vi "Failed attempt Main_11b.vi"() -> ()   [LabVIEW 2020]
uses:
  4985a7b0-beb7-44e5-b21a-1b7cc2dea417.vi
  Cluster_Multiply.ctl
panel:
  out "Array":T1(array[cluster])
  out "Answer":i32
  in  "Puzzle":string="Monkey 0:\n  Starting items: 72, 97\n  Operation: new = old * 13\n  Test: divisible by 19\n    If true: throw to monkey 5\n    If false: throw to monkey 6\n\nMonkey 1:\n  Starting items: 55, 70, 90, 74, 95\n  Operation: new = old * old\n  Test: divisible by 7\n    If true: throw to monkey 5\n    If false: throw to monkey 0\n\nMonkey 2:\n  Starting items: 74, 97, 66, 57\n  Operation: new = old + 6\n  Test: divisible by 17\n    If true: throw to monkey 1\n    If false: throw to monkey 0\n\nMonkey 3:\n  Starting items: 86, 54, 53\n  Operation: new = old + 2\n  Test: divisible by 13\n    If true: throw to monkey 1\n    If false: throw to monkey 2\n\nMonkey 4:\n  Starting items: 50, 65, 78, 50, 62, 99\n  Operation: new = old + 3\n  Test: divisible by 11\n    If true: throw to monkey 3\n    If false: throw to monkey 7\n\nMonkey 5:\n  Starting items: 90\n  Operation: new = old + 4\n  Test: divisible by 2\n    If true: throw to monkey 4\n    If false: throw to monkey 6\n\nMonkey 6:\n  Starting items: 88, 92, 63, 94, 96, 82, 53, 53\n  Operation: new = old + 8\n  Test: divisible by 5\n    If true: throw to monkey 4\n    If false: throw to monkey 7\n\nMonkey 7:\n  Starting items: 70, 60, 71, 69, 77, 70, 98\n  Operation: new = old * 7\n  Test: divisible by 3\n    If true: throw to monkey 2\n    If false: throw to monkey 3"
  in  "Example":string="Monkey 0:\n  Starting items: 79, 98\n  Operation: new = old * 19\n  Test: divisible by 23\n    If true: throw to monkey 2\n    If false: throw to monkey 3\n\nMonkey 1:\n  Starting items: 54, 65, 75, 74\n  Operation: new = old + 6\n  Test: divisible by 19\n    If true: throw to monkey 2\n    If false: throw to monkey 0\n\nMonkey 2:\n  Starting items: 79, 60, 97\n  Operation: new = old * old\n  Test: divisible by 13\n    If true: throw to monkey 1\n    If false: throw to monkey 3\n\nMonkey 3:\n  Starting items: 74\n  Operation: new = old + 3\n  Test: divisible by 17\n    If true: throw to monkey 0\n    If false: throw to monkey 1"
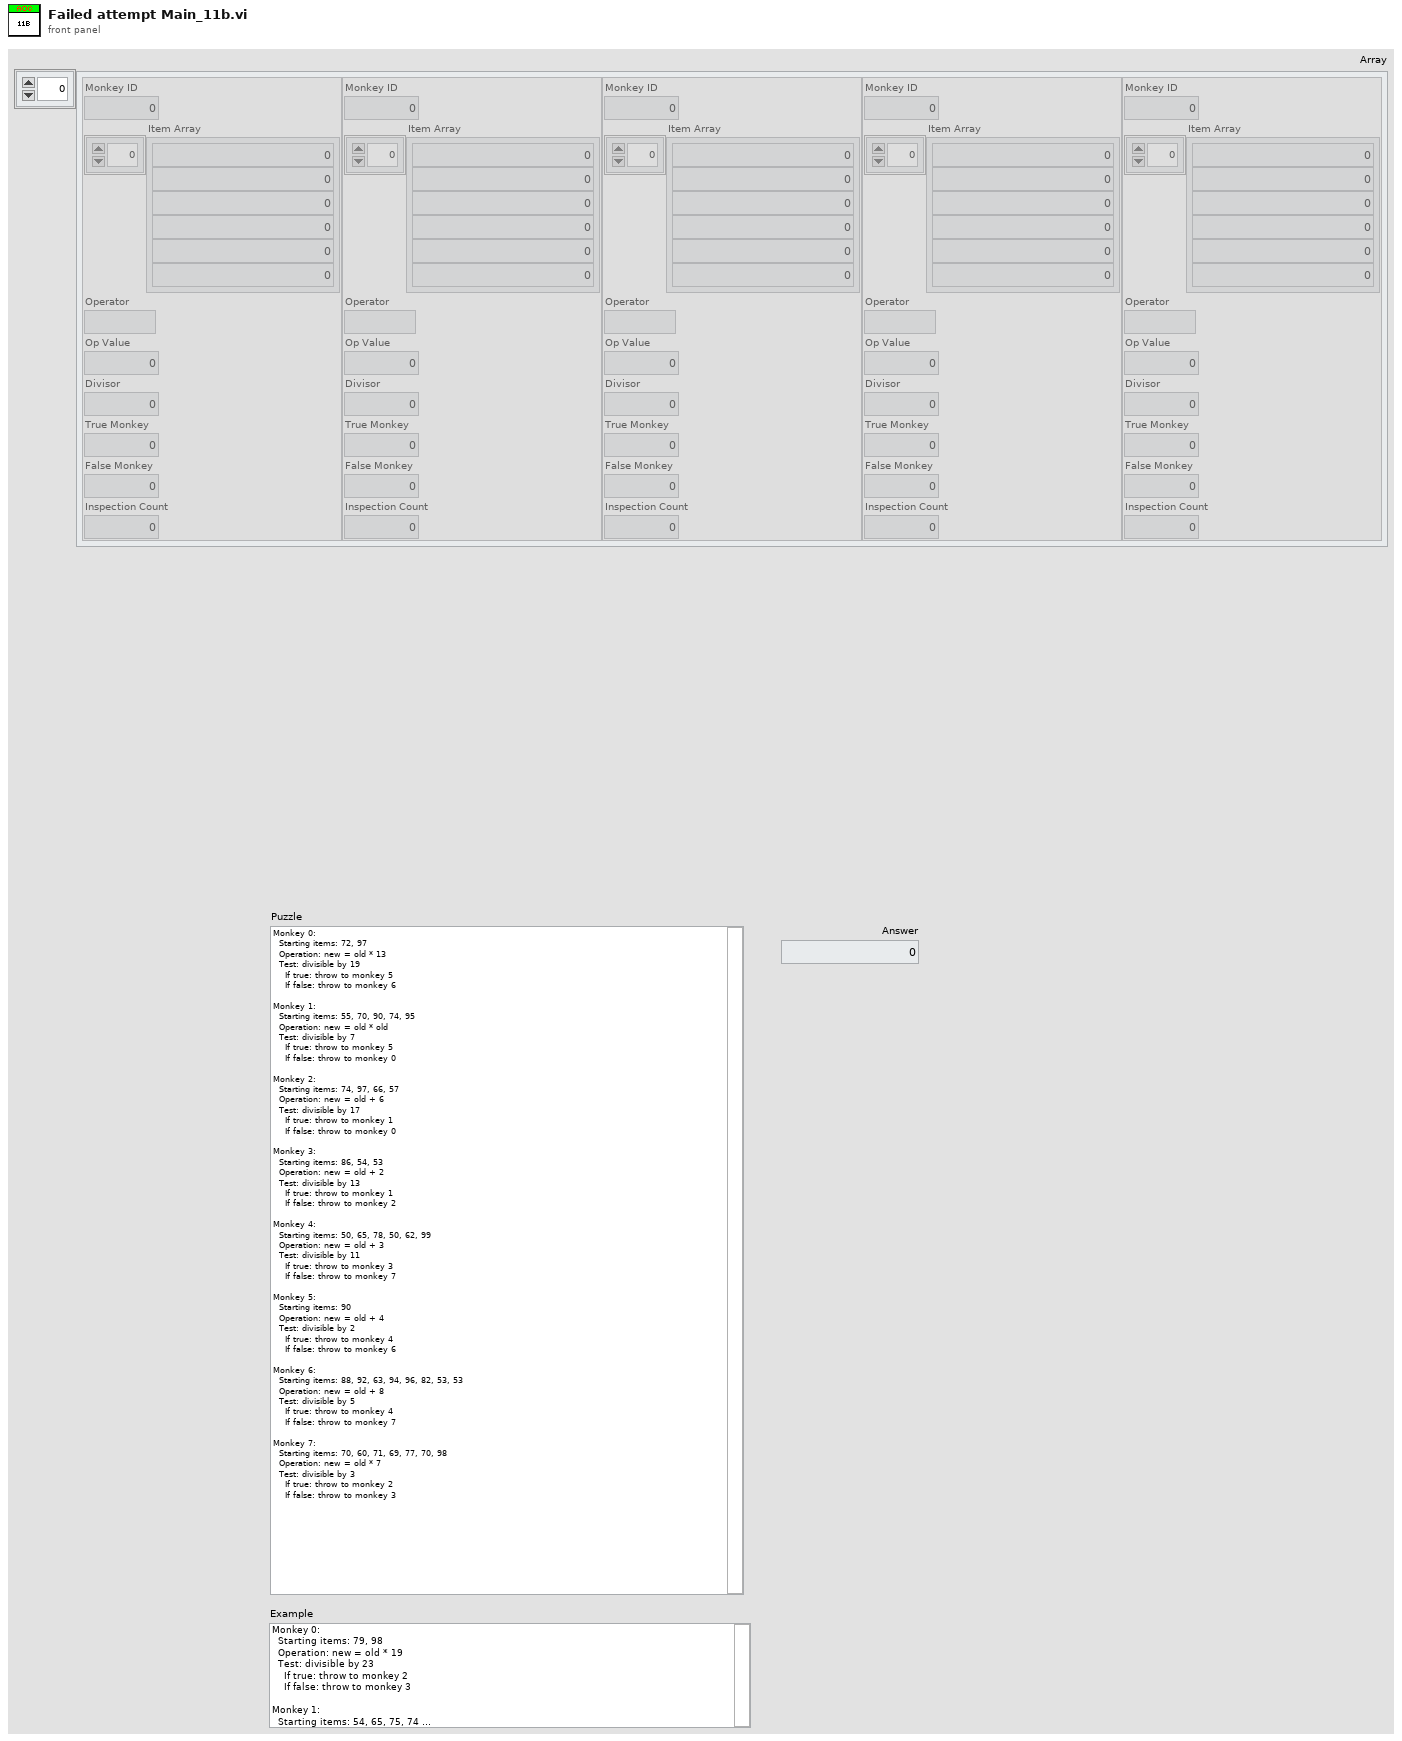
[diagram p1: front panel]
types:
  T1 = cluster{"Monkey ID":i32, "Item Array":u64[], "Operator":string, "Op Value":u64, "Divisor":u64, "True Monkey":i32, "False Monkey":i32, "Inspection Count":u64}[]
  T2 = typedef "Cluster_Multiply.ctl" = cluster{"Multiply Array":u64[]}
  T3 = cluster{"Monkey ID":i32, "Item":u64, "Operator":string, "Op Value":u64, "Divisor":u64, "True Monkey":i32, "False Monkey":i32, "Inspection Count":u64}
  T4 = cluster{"Monkey ID":i32, "Item":u64, "Operator":string, "Op Value":u64, "Divisor":u64, "True Monkey":i32, "False Monkey":i32, "Inspection Count":u64}[]
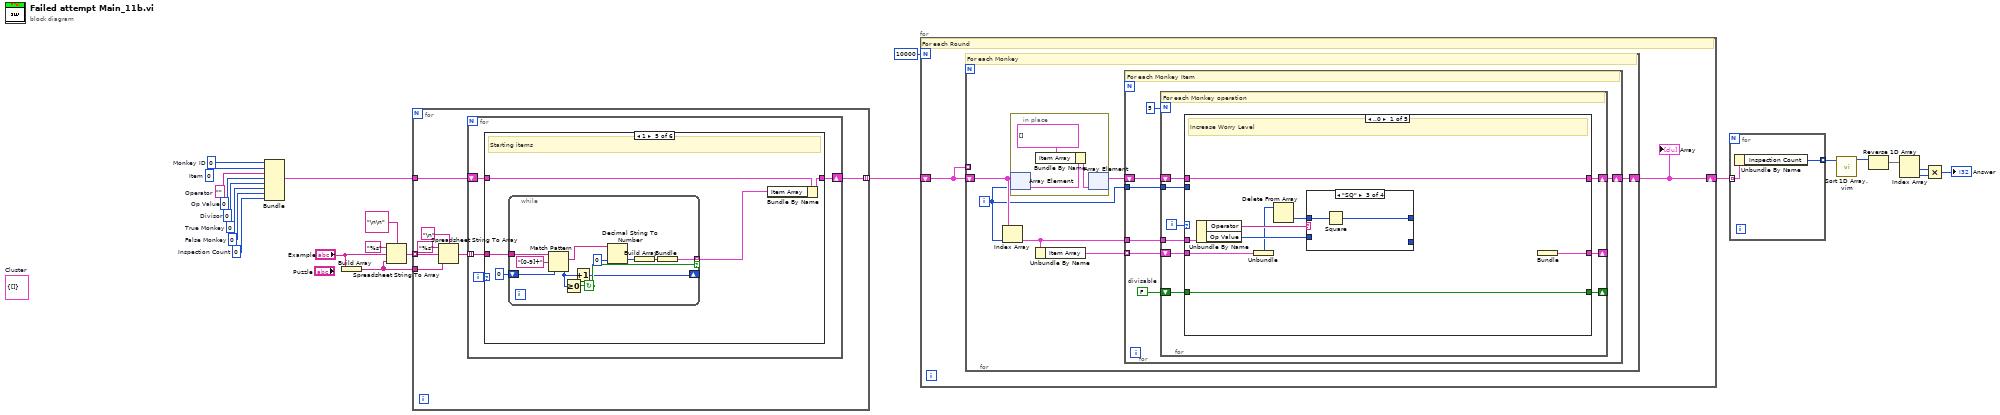
[diagram p0: block diagram]
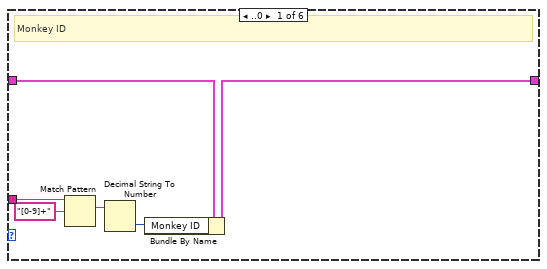
[diagram p2: hidden frame]
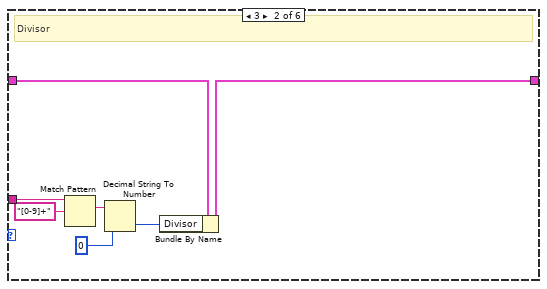
[diagram p3: hidden frame]
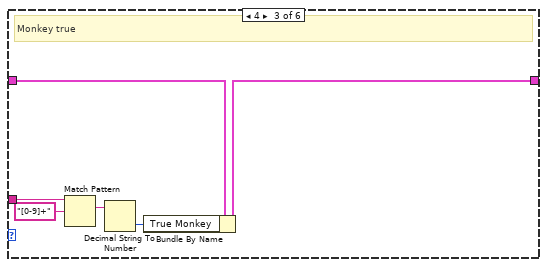
[diagram p4: hidden frame]
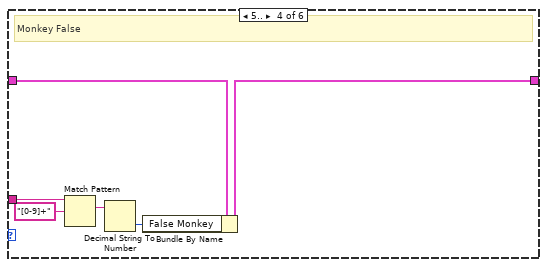
[diagram p5: hidden frame]
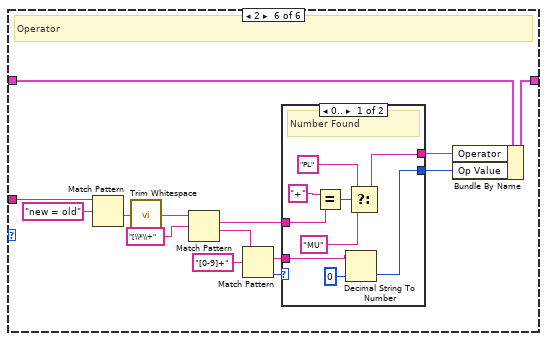
[diagram p6: hidden frame]
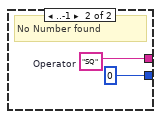
[diagram p7: hidden frame]
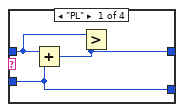
[diagram p8: hidden frame]
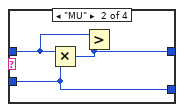
[diagram p9: hidden frame]
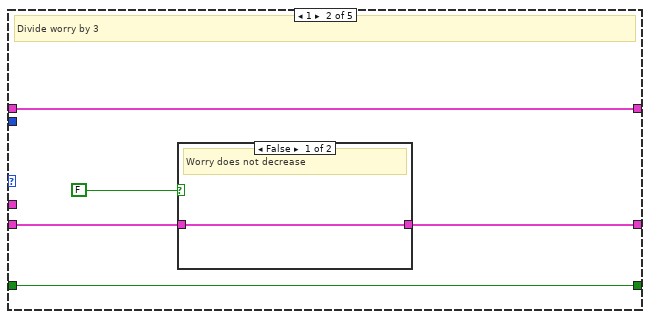
[diagram p11: hidden frame]
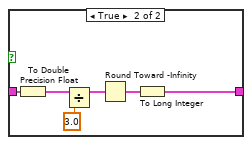
[diagram p12: hidden frame]
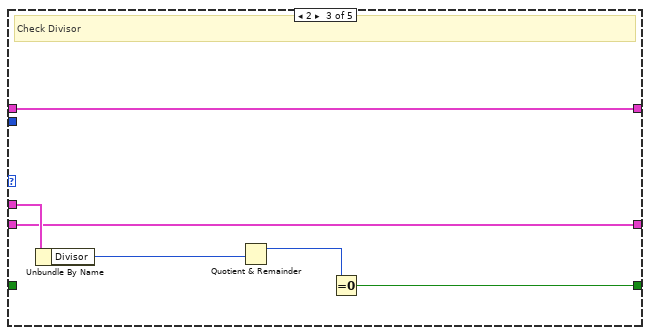
[diagram p13: hidden frame]
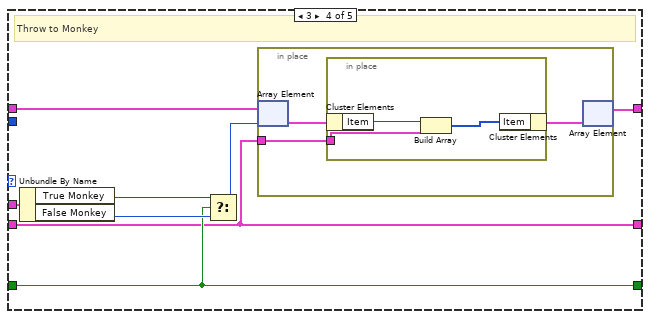
[diagram p14: hidden frame]
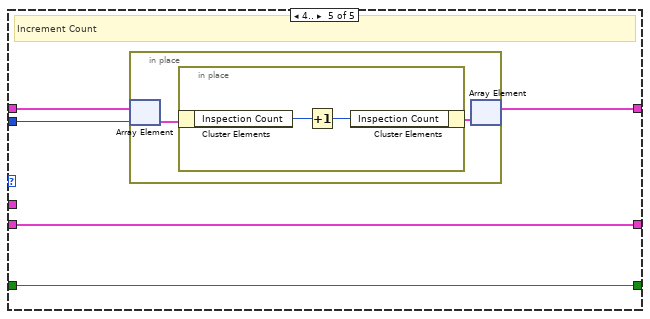
[diagram p15: hidden frame]
diagram:
  w1 = u64 0  # Item
  (unwired) T2 {"Multiply Array"=[]}  # Cluster
  w10 = u64 0  # Inspection Count
  w13 = 0  # False Monkey
  w14 = 0  # True Monkey
  w15 = u64 0  # Divisor
  w16 = u64 0  # Op Value
  w17 = ""  # Operator
  w18 = 0  # Monkey ID
  n1 = Bundle("Monkey ID"=w18, "Item"=w1, "Operator"=w17, "Op Value"=w16, "Divisor"=w15, "True Monkey"=w14, "False Monkey"=w13, "Inspection Count"=w10) -> (w12:T3)  [unwired: 1 in]
  n2 = Build Array("Example") -> (w19:string[])
  n3 = Spreadsheet String To Array(delimiter (Tab)="\n\n", format string="%s", spreadsheet string="Example", array type (2D Dbl)=w19) -> (array=w20:string[])
  n4 = for {
    tunnel: w20 -> [w30] mode=indexing
    tunnel: w19 -> [w27]
    tunnel: w12 -> [w25]
    tunnel: [w24] -> w11 mode=indexing
    n5 = Spreadsheet String To Array(delimiter (Tab)="\n", format string="%s", spreadsheet string=w30, array type (2D Dbl)=w27) -> (array=w26:string[])
    n6 = for {
      tunnel: w26 -> [w31] mode=indexing
      shift-right: [w32] -> w24
      shift-left: w25 -> [w33]
      i -> [w34]
      n7 = case shown="1" w34 {
        tunnel: w33 -> [w40 w47 w53 w59 w64 w89]
        tunnel: [w39 w46 w52 w58 w63 w88] -> w32
        tunnel: w31 -> [w38 w45 w51 w57 w62 w87]
        frame ..0 {
          # "Monkey ID"
          n8 = Match Pattern(string=w38, regular expression="[0-9]+") -> (match substring=w36:string)  [unwired: 1 in, 3 out]
          n9 = Decimal String To Number(string=w36) -> (number=w35:i32)  [unwired: 2 in, 1 out]
          n10 = Bundle By Name(cluster=w40, "Monkey ID"=w35) -> (w39:T3)
        }
        frame 3 {
          # "Divisor"
          n11 = Match Pattern(string=w45, regular expression="[0-9]+") -> (match substring=w43:string)  [unwired: 1 in, 3 out]
          n12 = Decimal String To Number(string=w43, default (0L)=u64 0 ("default (0 I32)")) -> (number=w42:u64)  [unwired: 1 in, 1 out]
          n13 = Bundle By Name(cluster=w47, "Divisor"=w42) -> (w46:T3)
        }
        frame 4 {
          # "Monkey true"
          n14 = Match Pattern(string=w51, regular expression="[0-9]+") -> (match substring=w49:string)  [unwired: 1 in, 3 out]
          n15 = Decimal String To Number(string=w49) -> (number=w48:i32)  [unwired: 2 in, 1 out]
          n16 = Bundle By Name(cluster=w53, "True Monkey"=w48) -> (w52:T3)
        }
        frame 5.. {
          # "Monkey False"
          n17 = Match Pattern(string=w57, regular expression="[0-9]+") -> (match substring=w55:string)  [unwired: 1 in, 3 out]
          n18 = Decimal String To Number(string=w55) -> (number=w54:i32)  [unwired: 2 in, 1 out]
          n19 = Bundle By Name(cluster=w59, "False Monkey"=w54) -> (w58:T3)
        }
        frame 1 {
          # "Starting items"
          n20 = while {
            tunnel: w62 -> [w75]
            tunnel: [w65] -> w60 mode=indexing if=w73
            shift-right: [w69] -> _
            shift-left: 0 -> [w68]
            stop <- w73 continue-if-true
            n21 = Match Pattern(string=w75, regular expression="[0-9]+", offset (0)=w68) -> (match substring=w72:string, offset past match=w70:i32)  [unwired: 2 out]
            n22 = Greater Or Equal To 0?(x=w70) -> (x >= 0?=w73:bool)
            n23 = Increment(x=w70) -> (x+1=w69:i32)
            n24 = Decimal String To Number(string=w72, default (0L)=u64 0 ("default (0 I32)")) -> (number=w71:u64)  [unwired: 1 in, 1 out]
            n25 = Build Array(w71) -> (w66:u64[])
            n26 = Bundle(w66) -> (w65:cluster{u64[]})  [unwired: 1 in]
          }
          n27 = Bundle By Name(cluster=w64, "Item Array"=w60) -> (w63:T3)
        }
        frame 2 {
          # "Operator"
          n28 = Match Pattern(string=w87, regular expression="new = old") -> (after substring=w85:string)  [unwired: 1 in, 3 out]
          n29 = call <vilib>:"Trim Whitespace.vi"("string"=w85) -> ("trimmed string"=w83:string)  [unwired: 1 in]
          n30 = Match Pattern(string=w83, regular expression="[\\*\\+") -> (match substring=w77:string, after substring=w82:string)  [unwired: 1 in, 2 out]
          n31 = Match Pattern(string=w82, regular expression="[0-9]+") -> (match substring=w76:string, offset past match=w80:i32)  [unwired: 1 in, 2 out]
          n32 = case shown="0.." w80 {
            tunnel: [w93 w100] -> w79
            tunnel: [w91 0] -> w78
            tunnel: w77 -> [w97 _]
            tunnel: w76 -> [w92 _]
            frame 0.. {
              # "Number Found"
              n33 = Equal?(x="+", y=w97) -> (x = y?=w96:bool)
              n34 = Decimal String To Number(string=w92, default (0L)=u64 0 ("default (0 I32)")) -> (number=w91:u64)  [unwired: 1 in, 1 out]
              n35 = Select(t="PL", s=w96, f="MU") -> (s? t:f=w93:string)
            }
            frame ..-1 {
              w100 = "SQ"  # Operator
              # "No Number found"
            }
          }
          n36 = Bundle By Name(cluster=w89, "Operator"=w79, "Op Value"=w78) -> (w88:T3)
        }
      }
    }
  }
  n37 = for {
    N: 10000 -> [_]
    shift-right: [w101] -> w9
    shift-left: w11 -> [w102]
    # "For each Round"
    n38 = for {
      shift-right: [w108] -> w101
      shift-left: w102 -> [w105]
      tunnel: w102 -> [_] mode=indexing
      i -> [w104]
      # "For each Monkey"
      n39 = Index Array(array=w105, index=w104) -> (element=w103:T3)
      n40 = in-place {
        n41 = in-place-array #1(w105, w104) -> (w111:T3)
        n42 = Bundle By Name(cluster=w111, "Item Array"=cluster{"Item Array":u64[]}[] []) -> (w110:T3)
        n43 = in-place-array #1(w110) -> (w106:T4)  [unwired: 1 out]
      }
      n44 = Unbundle By Name(w103) -> ("Item Array"=w107:T2[])
      n45 = for {
        tunnel: w103 -> [w116]
        tunnel: w107 -> [w117] mode=indexing
        shift-right: [w112] -> w108
        shift-left: w106 -> [w115]
        tunnel: w104 -> [w113]
        w114 = FALSE  # divisable
        # "For each Monkey Item"
        n46 = for {
          N: 5 -> [_]
          shift-right: [w123] -> _
          shift-left: w117 -> [w126]
          tunnel: w116 -> [w125]
          shift-right: [w122] -> w112
          shift-left: w115 -> [w124]
          shift-right: [w120] -> _
          shift-left: w114 -> [w121]
          tunnel: w113 -> [w119]
          i -> [w127]
          # "For each Monkey operation"
          n47 = case shown="..0" w127 {
            tunnel: w126 -> [w134 w153 w162 w167 w181]
            tunnel: w125 -> [w137 _ w165 w174 _]
            tunnel: w124 -> [w133 w151 w166 w170 w184]
            tunnel: [w130 w152 w162 w167 w181] -> w123
            tunnel: [w133 w151 w166 w169 w183] -> w122
            tunnel: w121 -> [w132 w150 _ w171 w185]
            tunnel: [w132 w150 w163 w171 w185] -> w120
            tunnel: w119 -> [_ _ _ _ w182]
            frame ..0 {
              # "Increase Worry Level"
              n48 = Unbundle By Name(w137) -> ("Operator"=w136:string, "Op Value"=w135:u64)
              n49 = Unbundle(w134) -> ("Multiply Array"=w128:u64[])
              n50 = Delete From Array(array=w128) -> (deleted portion=w131:u64)  [unwired: 2 in, 1 out]
              n51 = case shown="\"SQ\"" w136 {
                tunnel: w135 -> [w141 w145 _ _]
                tunnel: w131 -> [w140 w144 w146 w148]
                tunnel: [w139 w143 w147 w148] -> _
                tunnel: [w141 w145 _ _] -> _
                frame "PL" {
                  n52 = Add(x=w140, y=w141) -> (x+y=w139:u64)
                  n53 = Greater?(x=w140, y=w139) -> (0:w138:bool)
                }
                frame "MU" {
                  n54 = Multiply(x=w144, y=w145) -> (x*y=w143:u64)
                  n55 = Greater?(x=w144, y=w143) -> (0:w142:bool)
                }
                frame "SQ" {
                  n56 = Square(x=w146) -> (x^2=w147:u64)
                }
                frame Default {
                }
              }
              n57 = Bundle() -> (w130:cluster{void}, w129)  [unwired: 1 in]
            }
            frame 1 {
              # "Divide worry by 3"
              n58 = case shown="False" FALSE {
                tunnel: w153 -> [w154 w160]
                tunnel: [w154 w155] -> w152
                frame False {
                  # "Worry does not decrease"
                }
                frame True {
                  n59 = To Double Precision Float(number=w160) -> (double precision float=w159:cluster{"Multiply Array":dbl[]})
                  n60 = Divide(x=w159, y=3.0) -> (x/y=w157:cluster{"Multiply Array":dbl[]})
                  n61 = Round Toward -Infinity(1:w157) -> (0:w156:cluster{"Multiply Array":dbl[]})
                  n62 = To Long Integer(number=w156) -> (32bit integer=w155:cluster{"Multiply Array":i32[]})
                }
              }
            }
            frame 2 {
              # "Check Divisor"
              n63 = Unbundle By Name(w165) -> ("Divisor"=w164:u64)
              n64 = Quotient & Remainder(y=w164) -> (x-y*floor(x/y)=w161:u64)  [unwired: 1 in, 1 out]
              n65 = Equal To 0?(x=w161) -> (x = 0?=w163:bool)
            }
            frame 3 {
              # "Throw to Monkey"
              n66 = Unbundle By Name(w174) -> ("True Monkey"=w173:i32, "False Monkey"=w172:i32)
              n67 = Select(t=w173, s=w171, f=w172) -> (s? t:f=w168:i32)
              n68 = in-place {
                in-place-border: w167 -> [w175]
                n69 = in-place-array #2(w170, w168) -> (w177:T3)
                n70 = in-place {
                  in-place-border: w175 -> [w179]
                  n71 = in-place-cluster #3(w177) -> ("Item"=w180:u64)
                  n72 = Build Array(w180, w179) -> (w178:u64[])
                  n73 = in-place-cluster #3("Item"=w178) -> (w176:T3)
                }
                n74 = in-place-array #2(w176) -> (w169:T4)  [unwired: 1 out]
              }
            }
            frame 4.. {
              # "Increment Count"
              n75 = in-place {
                n76 = in-place-array #4(w184, w182) -> (w187:T3)
                n77 = in-place {
                  n78 = in-place-cluster #5(w187) -> ("Inspection Count"=w189:u64)
                  n79 = Increment(x=w189) -> (x+1=w188:u64)
                  n80 = in-place-cluster #5("Inspection Count"=w188) -> (w186:T3)
                }
                n81 = in-place-array #4(w186) -> (w183:T4)  [unwired: 1 out]
              }
            }
          }
        }
      }
    }
    "Array" <- w101
  }
  n82 = for {
    tunnel: w9 -> [w191] mode=indexing
    tunnel: [w190] -> w8 mode=indexing
    n83 = Unbundle By Name(w191) -> ("Inspection Count"=w190:u64)
  }
  n84 = call "Sort 1D Array.vim"("unsorted array"=w8) -> ("sorted array"=w7:u64[])  [unwired: 10 in]
  n85 = Reverse 1D Array(array=w7) -> (reversed array=w6:u64[])
  n86 = Index Array(array=w6) -> (element #1=w4:u64, element #2=w5:u64)  [unwired: 2 in]
  n87 = Multiply(x=w4, y=w5) -> (x*y=→"Answer":u64)
